vi "Close Dut.vi"(8 "error in (no error)":errorcluster, 11 "_hResourceContext":u32) -> (0 "error out":errorcluster, 2 "function return":bool, 3 "_hResourceContext out":u32)   [LabVIEW 2013, in "QCAWLAN_DLL.lvlib"]
doc: "QCA_DLL_Export bool CloseDut(HANDLE _hResourceContext);"
uses:
  QCAWLAN_DLL.lvlib
  QCAWLAN_DLL.dll
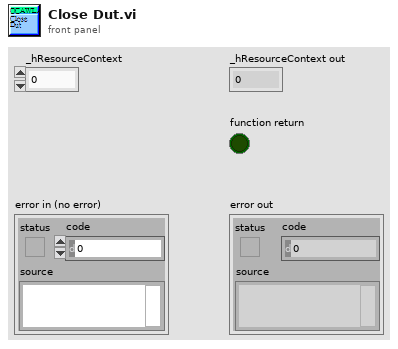
[diagram p1: front panel]
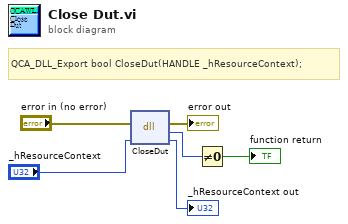
[diagram p0: block diagram]
diagram:
  # "QCA_DLL_Export bool CloseDut(HANDLE _hResourceContext);"
  n1 = dll-call lib="C:/Connectivity Client - MIMO/PlugIn/QCAWLAN_DLL.*" fn="CloseDut"(error in="error in (no error)", "_hResourceContext"="_hResourceContext") -> (error out=→"error out":errorcluster, w5:u8, "_hResourceContext"=→"_hResourceContext out":u32)  [unwired: 2 in, 1 out]
  n2 = Not Equal To 0?(x=w5) -> (x != 0?=→"function return":bool)
